vi "stepTrigger.vi"(0 "triggerReadout":u16) -> (14 "triggeredScan":bool)   [LabVIEW 2014]
uses:
  Sequencer/sequencerGlobVars.vi
  stepTriggerGlobalVars.vi
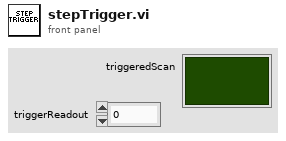
[diagram p1: front panel]
types:
  T1 = typedef "triggerTypes.ctl" = enum16{"noTrigger", "singleHitDelay", "singleHit", "software", "sweep"}
  T2 = typedef "selectTrigger.ctl" = enum8{"Ext0", "Ext1", "Ext2", "Ext3", "Ext4", "Ext5", "Ext6", "Ext7", "Int0", "Int1", "Int2", "Int3", "Int4", "Int5", "Int6", "Int7"}
  T3 = typedef "triggerEdge.ctl" = enum8{"either", "false-true", "true-false"}
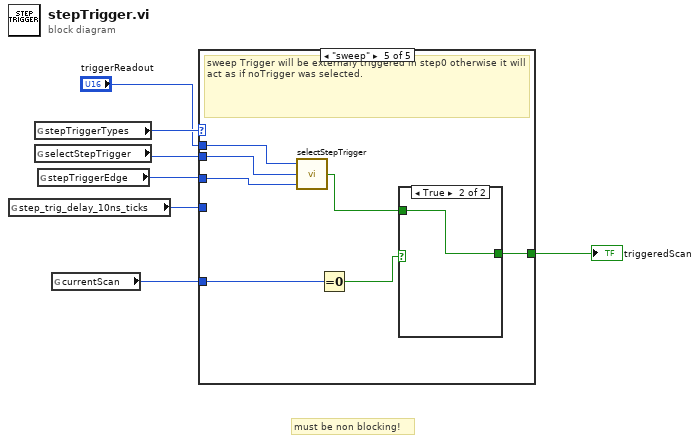
[diagram p0: block diagram]
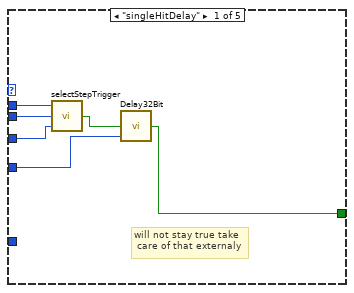
[diagram p2: hidden frame]
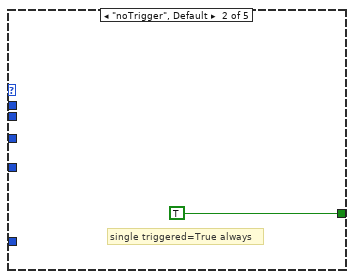
[diagram p3: hidden frame]
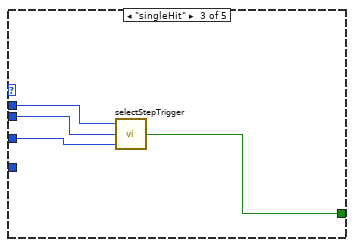
[diagram p4: hidden frame]
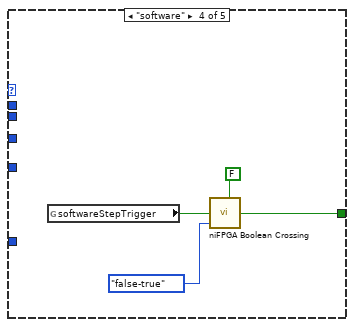
[diagram p5: hidden frame]
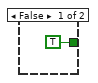
[diagram p6: hidden frame]
diagram:
  # "must be non blocking!"
  n1 = global read "stepTriggerGlobalVars.vi" "step_trig_delay_10ns_ticks"() -> (w2:u32)
  n2 = global read "stepTriggerGlobalVars.vi" "stepTriggerTypes"() -> (w5:T1)
  n3 = global read "stepTriggerGlobalVars.vi" "selectStepTrigger"() -> (w4:T2)
  n4 = global read "stepTriggerGlobalVars.vi" "stepTriggerEdge"() -> (w3:T3)
  n5 = global read "sequencerGlobVars.vi" "currentScan"() -> (w6:i32)
  n6 = case shown="\"sweep\"" w5 {
    tunnel: w4 -> [w11 _ w17 _ w25]
    tunnel: w2 -> [w13 _ _ _ _]
    tunnel: [w12 TRUE w18 w22 w27] -> w7
    tunnel: w3 -> [w10 _ w16 _ w24]
    tunnel: w6 -> [_ _ _ _ w29]
    tunnel: "triggerReadout" -> [w8 _ w15 _ w23]
    frame "singleHitDelay" {
      # "will not stay true take\n care of that externaly"
      n7 = call "selectStepTrigger.vi"("stepTriggerEdge"=w10, "MCSSelectStepTrigger"=w11, "triggerReadout"=w8) -> ("fired"=w9:bool)  [unwired: 2 in]
      n8 = call "Delay32Bit.vi"("delay(ticks)"=w13, "In"=w9) -> ("Out"=w12:bool)  [unwired: 3 in]
    }
    frame "noTrigger", Default {
      # "single triggered=True always"
    }
    frame "singleHit" {
      n9 = call "selectStepTrigger.vi"("stepTriggerEdge"=w16, "MCSSelectStepTrigger"=w17, "triggerReadout"=w15) -> ("fired"=w18:bool)  [unwired: 2 in]
    }
    frame "software" {
      n10 = global read "stepTriggerGlobalVars.vi" "softwareStepTrigger"() -> (w19:bool)
      n11 = call <vilib>:"niFPGA Boolean Crossing.vi"("input"=w19, "direction"=enum8{"either", "false-true", "true-false"}."false-true", "initialize"=FALSE) -> ("crossing"=w22:bool)  [unwired: 6 in]
    }
    frame "sweep" {
      # "sweep Trigger will be externaly triggered in step0 otherwise it will act as if noTrigger was selected."
      n12 = call "selectStepTrigger.vi"("stepTriggerEdge"=w24, "MCSSelectStepTrigger"=w25, "triggerReadout"=w23) -> ("fired"=w26:bool)  [unwired: 2 in]
      n13 = Equal To 0?(x=w29) -> (x = 0?=w28:bool)
      n14 = case shown="True" w28 {
        tunnel: w26 -> [_ w31]
        tunnel: [TRUE ("fired") w31] -> w27
        frame False {
        }
        frame True {
        }
      }
    }
  }
  "triggeredScan" <- w7
